vi "Filter and trim data.vi"(9 "q Starting":dbl, 10 "q Final":dbl, 11 "Data":cluster{"Angle":dbl, "Data":dbl}[](array[cluster])) -> (1 "New intensity arr":dbl[](array[numeric]), 2 "New angle arr":dbl[](array[numeric]), 3 "SPR curve":cluster{"Angle":dbl, "Data":dbl}[](array[cluster]))   [LabVIEW 2020]
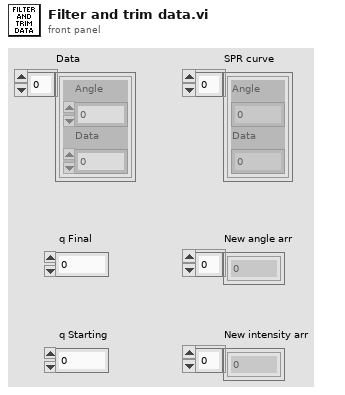
[diagram p1: front panel]
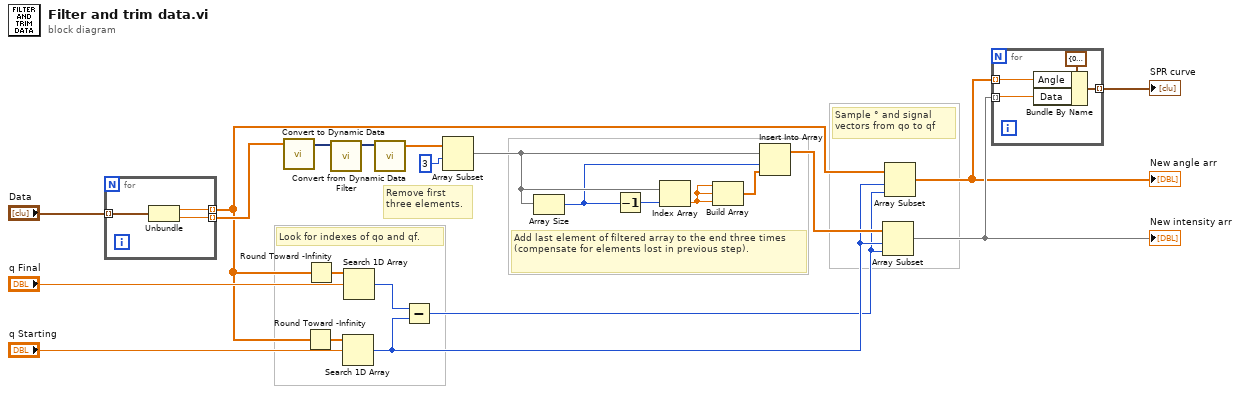
[diagram p0: block diagram]
diagram:
  # "Sample ° and signal vectors from qo to qf"
  # "Add last element of filtered array to the end three times (compensate for elements lost in previous step)."
  # "Remove first three elements."
  # "Look for indexes of qo and qf."
  n1 = for {
    tunnel: "Data" -> [w26] mode=indexing
    tunnel: [w25] -> w6 mode=indexing
    tunnel: [w24] -> w23 mode=indexing
    n2 = Unbundle(w26) -> ("Angle"=w25:dbl, "Data"=w24:dbl)
  }
  n3 = call "Convert to Dynamic Data"("Array"=w23) -> ("Dynamic Data Type"=w20:dynamicdata)  [unwired: 3 in]
  n4 = Round Toward -Infinity(1:w6) -> (0:w8:dbl[])
  n5 = Round Toward -Infinity(1:w6) -> (0:w9:dbl[])
  n6 = call "Filter"("Signal"=w20) -> ("Filtered Signal"=w19:dynamicdata)  [unwired: 9 in, 1 out]
  n7 = Search 1D Array(1D array=w8, element="q Starting") -> (index of element=w5:i32)  [unwired: 1 in]
  n8 = Search 1D Array(1D array=w9, element="q Final") -> (index of element=w21:i32)  [unwired: 1 in]
  n9 = call "Convert from Dynamic Data"("Dynamic Data Type"=w19) -> ("Array"=w12:dbl[])  [unwired: 3 in]
  n10 = Subtract(x=w21, y=w5) -> (x-y=w4:i32)
  n11 = Array Subset(array=w12, index=3 ("length")) -> (w17:dbl[])  [unwired: 1 in]
  n12 = Array Size(array=w17) -> (size(s)=w14:i32)
  n13 = Decrement(x=w14) -> (x-1=w16:i32)
  n14 = Index Array(array=w17, index=w16) -> (element=w15:dbl)
  n15 = Build Array(w15, w15, w15) -> (w13:dbl[])
  n16 = Insert Into Array(array=w17, index=w14, new element=w13) -> (w7:dbl[])
  n17 = Array Subset(array=w7, index=w5, length=w4) -> (w3:dbl[])
  "New intensity arr" <- w3
  n18 = Array Subset(array=w6, index=w5, length=w4) -> (w2:dbl[])
  "New angle arr" <- w2
  n19 = for {
    tunnel: w2 -> [w29] mode=indexing
    tunnel: [w28] -> w1 mode=indexing
    tunnel: w3 -> [w27] mode=indexing
    n20 = Bundle By Name(cluster=cluster{"Angle":dbl, "Data":dbl} {"Angle"=0.0, "Data"=0.0} ("Angle vs V"), "Angle"=w29, "Data"=w27) -> (w28:cluster{"Angle":dbl, "Data":dbl})
  }
  "SPR curve" <- w1
